vi "GEA2 Script_Dequeue Stop.vi"(11 "error in (no error)":errorcluster) -> (4 "Stop Queue?":bool, 15 "error out":errorcluster)   [LabVIEW 2023]
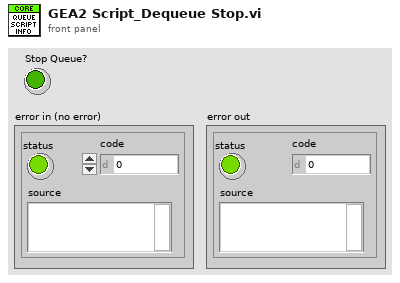
[diagram p1: front panel]
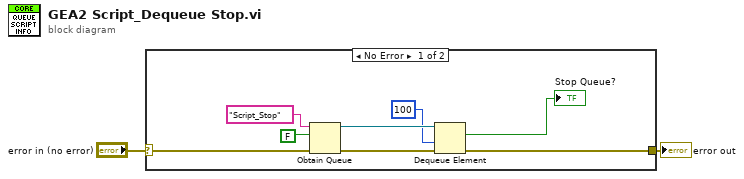
[diagram p0: block diagram]
diagram:
  n1 = case shown="No Error" "error in (no error)" {
    selector: "error in (no error)" -> [w10 w11]
    tunnel: [w3 w11] -> w2
    frame No Error {
      n2 = Obtain Queue(name (unnamed)="Script_Stop", element data type=FALSE, error in (no error)=w10) -> (queue out=w8:refnum<queue>, error out=w9:errorcluster)  [unwired: 2 in, 1 out]
      n3 = Dequeue Element(queue=w8, timeout in ms (-1)=100, error in (no error)=w9) -> (element=→"Stop Queue?":bool, error out=w3:errorcluster)  [unwired: 2 out]
    }
    frame Error {
    }
  }
  "error out" <- w2
